vi "Brocast Data.vi"(8 "error in (no error)":errorcluster, 9 "Models Enqueue.lvclass":refnum<class "Enqueues Data.lvclass">, 10 "Views Enqueue.lvclass":refnum<class "Enqueues Data.lvclass">, 11 "MVVM Abstruct Model in":refnum<class "MVVM Abstruct Model.lvclass">) -> (0 "error out":errorcluster, 3 "MVVM Abstruct Model out":refnum<class "MVVM Abstruct Model.lvclass">)   [LabVIEW 2020, in "MVVM Abstruct Model.lvlib" / "MVVM Abstruct Model.lvclass"]
uses:
  MVVM Abstruct Model.lvclass
  Enqueues Data/Enqueues Data.lvclass
  Enqueues Data/Enqueues Data.lvclass/Enqueues Data.ctl
  MVVM Abstruct Model.lvclass/MVVM Abstruct Model.ctl
  Enqueues Data/Accessors/Read ActorMap.vi
  C:/Users/yu/Desktop/Pro1/06 Source/Code/Common/ActorMap/ActorMap.lvclass
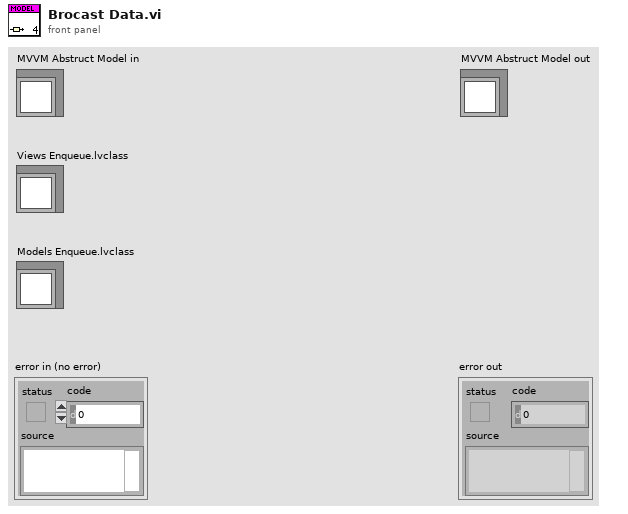
[diagram p1: front panel]
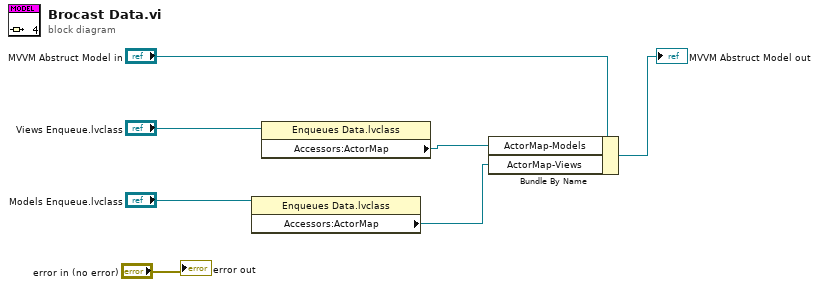
[diagram p0: block diagram]
diagram:
  n1 = property class="Enqueues Data.lvclass"(reference="Models Enqueue.lvclass") -> ("Accessors:ActorMap"=w3:refnum<class "ActorMap.lvclass">)  [unwired: 1 in, 2 out]
  n2 = property class="Enqueues Data.lvclass"(reference="Views Enqueue.lvclass") -> ("Accessors:ActorMap"=w4:refnum<class "ActorMap.lvclass">)  [unwired: 1 in, 2 out]
  n3 = Bundle By Name(cluster="MVVM Abstruct Model in", "ActorMap-Models"=w4, "ActorMap-Views"=w3) -> (→"MVVM Abstruct Model out":refnum<class "MVVM Abstruct Model.lvclass">)
  "error out" <- "error in (no error)"
